vi "ARRET.vi"(11 "arrêt":bool) -> (3 "T button?":bool)   [LabVIEW 2020]
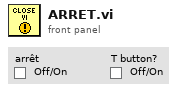
[diagram p1: front panel]
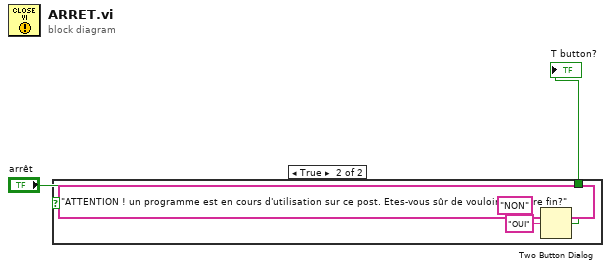
[diagram p0: block diagram]
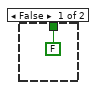
[diagram p2: hidden frame]
diagram:
  n1 = case shown="True" "arrêt" {
    tunnel: [FALSE ("T button?") w7] -> w2
    frame False {
    }
    frame True {
      n2 = Two Button Dialog(message="ATTENTION ! un programme est en cours d'utilisation sur ce post. Etes-vous sûr de vouloir y mettre fin?", 1:"NON" ("Nom du bouton F (\"Annuler\")"), 2:"OUI" ("Nom du bouton V (\"OK\")")) -> (T button?=w7:bool)
    }
  }
  "T button?" <- w2
